vi "update_exp_state.vi"(8 "ERROR IN":errorcluster, 10 "NEW STATE":T1, 11 "EXP SETTINGS":refnum<notifier>) -> (0 "ERROR OUT":errorcluster, 3 "EXP SETTINGS UPDATED":refnum<notifier>)   [LabVIEW 2013]
uses:
  type_defs/experiment_settings.ctl
  type_defs/experiment_states.ctl
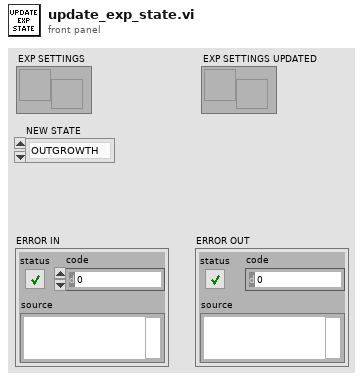
[diagram p1: front panel]
types:
  T1 = typedef "experiment_states.ctl" = enum16{"OUTGROWTH", "INDUCTION", "EXPERIMENT"}
  T2 = typedef "experiment_settings.ctl" = cluster{"fcs file byte offset":i64, "LED Device Handle Out":u32, "START TIME":timestamp, "CURRENT VALVE":u32, "SAMPLE #":i32, "FCS FILE PATH":path, "TIME POINT":i32, "STATE":T1, "TIME TILL SAMPLE":dbl, "DILUTION  TABLE":dbl[][]}
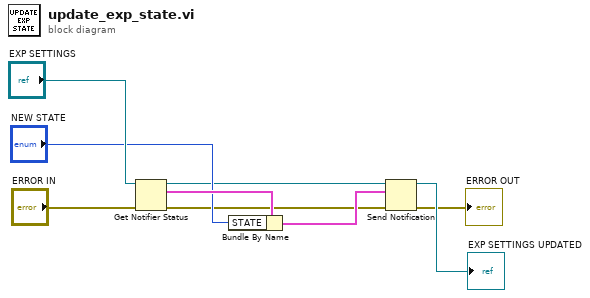
[diagram p0: block diagram]
diagram:
  n1 = Get Notifier Status(notifier="EXP SETTINGS", error in (no error)="ERROR IN") -> (notifier out=w3:refnum<notifier>, current notification=w7:T2, error out=w4:errorcluster)  [unwired: 2 out]
  n2 = Bundle By Name(cluster=w7, "STATE"="NEW STATE") -> (w6:T2)
  n3 = Send Notification(notification=w6, notifier=w3, error in (no error)=w4) -> (notifier out=→"EXP SETTINGS UPDATED":refnum<notifier>, error out=→"ERROR OUT":errorcluster)
